vi "Varian Magnet Scan.vi"(8 "error in (no error)":errorcluster, 10 "Varian Magnet.lvclass":refnum<class "Varian Magnet.lvclass">, 11 "Varian Magnet Scan in":refnum<class "Varian Magnet Scan.lvclass">) -> (0 "error out":errorcluster, 3 "Varian Magnet Scan out":refnum<class "Varian Magnet Scan.lvclass">)   [LabVIEW 2009, in "Varian Magnet Scan.lvclass"]
uses:
  Varian Magnet Scan.lvclass
  Instruments/Varian Magnet/Varian Magnet.lvclass
  Scanner/Scanner.lvclass
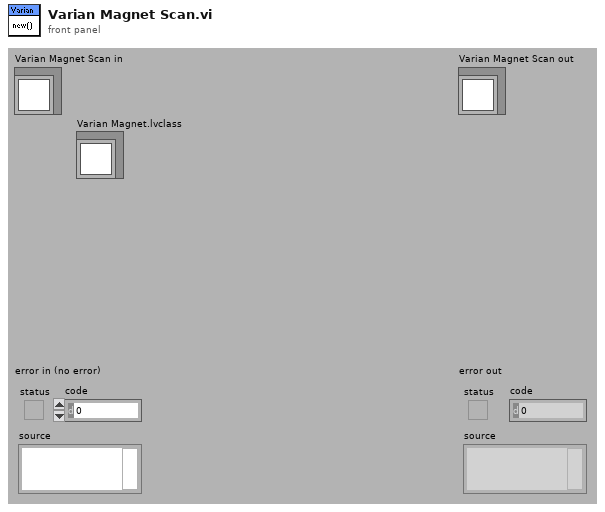
[diagram p1: front panel]
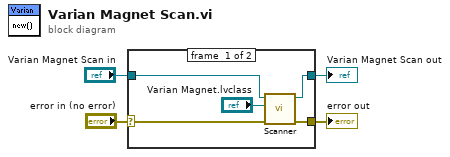
[diagram p0: block diagram]
diagram:
  n1 = case shown="No Error" "error in (no error)" {
    selector: "error in (no error)" -> [w7 w11]
    tunnel: [w6 w11] -> w3
    tunnel: [w8 w10] -> w1
    tunnel: "Varian Magnet Scan in" -> [w9 w10]
    frame #0 {
      n2 = call "Scanner.vi"("error in (no error)"=w7, "Scannable"="Varian Magnet.lvclass", "Scanner.lvclass in"=w9) -> ("error out"=w6:errorcluster, "Scanner.lvclass out"=w8:refnum<class "Varian Magnet Scan.lvclass">)  [unwired: 1 in, 6 out]
    }
    frame #1 {
    }
  }
  "error out" <- w3
  "Varian Magnet Scan out" <- w1
